vi "Filter - tag prefix.vi"(8 "error in (no error)":errorcluster) -> (0 "error out":errorcluster)   [LabVIEW 2026, in "Tests.lvlib"]
doc: "Unit test (Caraya). Verifies RoutedFilterMatch tag-prefix matching on a dot-hierarchy boundary: an exact tag and a child tag match, a sibling that merely shares a textual prefix does not, and an empty prefix matches any (SRS-LMBR-027). Level is held within the band so acceptance depends only on the tag. Pure, no fixtures. The routed level-range behavior is covered separately."
uses:
  Tests.lvlib
  src/TypeDefs/Statement.ctl
  src/TypeDefs/Severity.ctl
  src/TypeDefs/Filter.ctl
  src/TypeDefs/FilterMode.ctl
  <vilib>/addons/_JKI Toolkits/Caraya/classes/Assert/Assert True.vi
  <vilib>/addons/_JKI Toolkits/Caraya/classes/Assert/Assert False.vi
  <vilib>/addons/_JKI Toolkits/Caraya/classes/Test/Test.lvclass
  <vilib>/addons/_JKI Toolkits/Caraya/classes/Assert/Assert.lvclass
  src/Lumberjack.lvlib
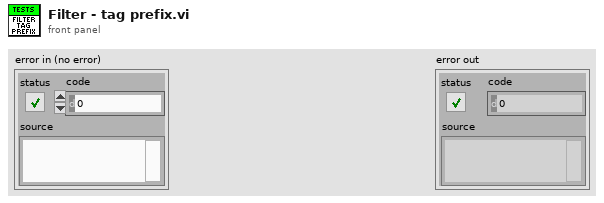
[diagram p1: front panel]
types:
  T1 = typedef "Lumberjack.lvlib/Severity.ctl" = enum16{"OFF", "FATAL", "ERROR", "WARN", "INFO", "DEBUG", "TRACE", "ALL"}
  T2 = typedef "Lumberjack.lvlib/Filter.ctl" = cluster{"mode":T3, "levelMin":T1, "levelMax":T1, "tagPrefix":string}
  T3 = typedef "Lumberjack.lvlib/FilterMode.ctl" = enum16{"Mirror", "Routed"}
  T4 = typedef "Lumberjack.lvlib/Statement.ctl" = cluster{"timestamp":timestamp, "level":T1, "sourceTag":string, "originVI":string, "message":string}
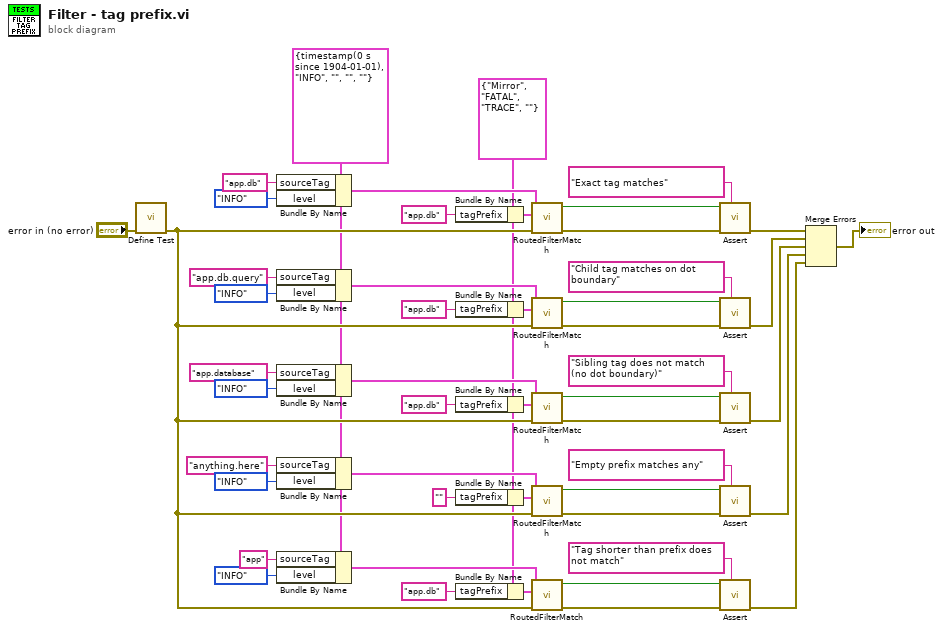
[diagram p0: block diagram]
diagram:
  w10 = T2 {"mode"=enum."Mirror", "levelMin"=enum."FATAL", "levelMax"=enum."TRACE", "tagPrefix"=""} ("Filter")
  w11 = T4 {"timestamp"=timestamp(0 s since 1904-01-01), "level"=enum."INFO", "sourceTag"="", "originVI"="", "message"=""} ("Statement")
  n1 = call <vilib>:"Define Test.vi"("error in (no error)"="error in (no error)") -> ("error out"=w12:errorcluster)  [unwired: 9 in, 1 out]
  n2 = Bundle By Name(cluster=w11, "sourceTag"="app.db", "level"=Severity."INFO") -> (w46:T4)
  n3 = Bundle By Name(cluster=w11, "sourceTag"="app.db.query", "level"=Severity."INFO") -> (w39:T4)
  n4 = Bundle By Name(cluster=w11, "sourceTag"="app.database", "level"=Severity."INFO") -> (w32:T4)
  n5 = Bundle By Name(cluster=w11, "sourceTag"="anything.here", "level"=Severity."INFO") -> (w25:T4)
  n6 = Bundle By Name(cluster=w11, "sourceTag"="app", "level"=Severity."INFO") -> (w18:T4)
  n7 = Bundle By Name(cluster=w10, "tagPrefix"="app.db") -> (w42:T2)
  n8 = Bundle By Name(cluster=w10, "tagPrefix"="app.db") -> (w35:T2)
  n9 = Bundle By Name(cluster=w10, "tagPrefix"="app.db") -> (w28:T2)
  n10 = Bundle By Name(cluster=w10, "tagPrefix"="") -> (w21:T2)
  n11 = Bundle By Name(cluster=w10, "tagPrefix"="app.db") -> (w14:T2)
  n12 = call "RoutedFilterMatch.vi"("error in (no error)"=w12, "Filter"=w42, "Statement"=w46) -> ("error out"=w47:errorcluster, "Accepted"=w43:bool)  [unwired: 7 in]
  n13 = call "RoutedFilterMatch.vi"("error in (no error)"=w12, "Filter"=w35, "Statement"=w39) -> ("error out"=w40:errorcluster, "Accepted"=w36:bool)  [unwired: 7 in]
  n14 = call "RoutedFilterMatch.vi"("error in (no error)"=w12, "Filter"=w28, "Statement"=w32) -> ("error out"=w33:errorcluster, "Accepted"=w29:bool)  [unwired: 7 in]
  n15 = call "RoutedFilterMatch.vi"("error in (no error)"=w12, "Filter"=w21, "Statement"=w25) -> ("error out"=w26:errorcluster, "Accepted"=w22:bool)  [unwired: 7 in]
  n16 = call "RoutedFilterMatch.vi"("error in (no error)"=w12, "Filter"=w14, "Statement"=w18) -> ("error out"=w19:errorcluster, "Accepted"=w15:bool)  [unwired: 7 in]
  n17 = call-poly <vilib>:"Assert.vi"("Label"="Exact tag matches", "error in (no error)"=w47, "True?"=w43) -> ("error out"=w48:errorcluster)  [unwired: 7 in, 1 out]
  n18 = call-poly <vilib>:"Assert.vi"("Label"="Child tag matches on dot boundary", "error in (no error)"=w40, "True?"=w36) -> ("error out"=w9:errorcluster)  [unwired: 7 in, 1 out]
  n19 = call-poly <vilib>:"Assert.vi"("Label"="Sibling tag does not match (no dot boundary)", "error in (no error)"=w33, "False?"=w29) -> ("error out"=w8:errorcluster)  [unwired: 7 in, 1 out]
  n20 = call-poly <vilib>:"Assert.vi"("Label"="Empty prefix matches any", "error in (no error)"=w26, "True?"=w22) -> ("error out"=w7:errorcluster)  [unwired: 7 in, 1 out]
  n21 = call-poly <vilib>:"Assert.vi"("Label"="Tag shorter than prefix does not match", "error in (no error)"=w19, "False?"=w15) -> ("error out"=w6:errorcluster)  [unwired: 7 in, 1 out]
  n22 = Merge Errors(w48, w9, w8, w7, w6) -> (→"error out":errorcluster)
